vi "write_cred_xml.vi"() -> ()   [LabVIEW 2018]
uses:
  Ctrl/cred_ctrl.ctl
  Ctrl/cred_ip_info.ctl
  Ctrl/data_cred.ctl
  DataBase/MYsql/lv_mysql_connector_v1_lv8/typedefs/mysql_authentication.ctl
  <vilib>/NI/GXML/GXML.lvlib
panel:
  in  "database_inf":T1
  in  "database_ip":T2
  out "error out":errorcluster
  in  "XML File Path":path=path "C:/Users/prone/OneDrive/Documents/Acquire_MAP_copy-master/Acquire_MAP_copy-master/ignore/creds.xml"
  in  "error in":errorcluster
  in  "storage":T4
  out "XML String Out":string
  in  "slack":T4
  in  "database":T4
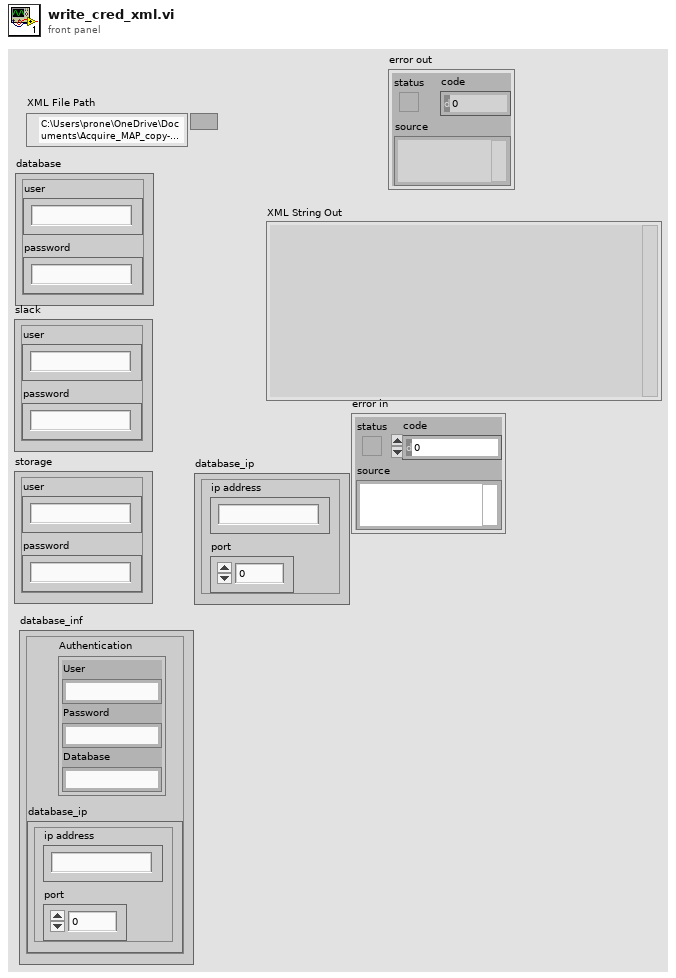
[diagram p1: front panel]
types:
  T1 = typedef "data_cred.ctl" = cluster{"database_ip":T2, "Authentication":T3}
  T2 = typedef "cred_ip_info.ctl" = cluster{"ip address":string, "port":dbl}
  T3 = typedef "mysql_authentication.ctl" = cluster{"User":string, "Password":string, "Database":string}
  T4 = typedef "cred_ctrl.ctl" = cluster{"user":string, "password":string}
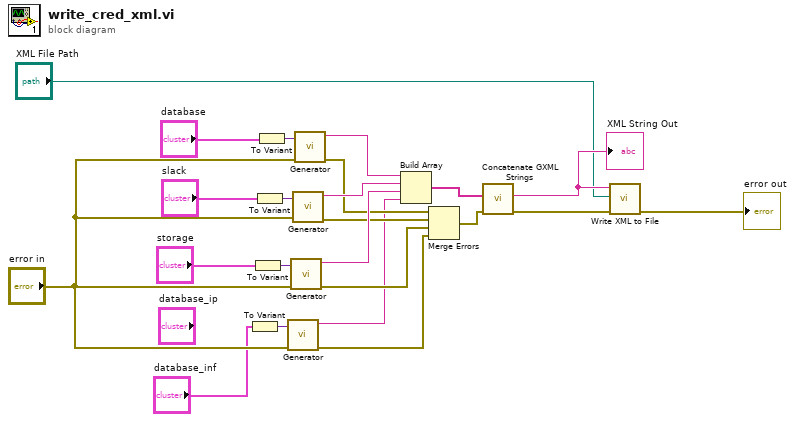
[diagram p0: block diagram]
diagram:
  n1 = To Variant(anything="database_inf") -> (Variant=w5:variant)
  n2 = To Variant(anything="storage") -> (Variant=w16:variant)
  n3 = To Variant(anything="slack") -> (Variant=w21:variant)
  n4 = To Variant(anything="database") -> (Variant=w23:variant)
  n5 = call <vilib>:"Generator.vi"("error in"="error in", "Variant"=w5) -> ("error out"=w3:errorcluster, "XML String Out"=w2:string)  [unwired: 8 in]
  n6 = call <vilib>:"Generator.vi"("error in"="error in", "Variant"=w16) -> ("error out"=w11:errorcluster, "XML String Out"=w14:string)  [unwired: 8 in]
  n7 = call <vilib>:"Generator.vi"("error in"="error in", "Variant"=w21) -> ("error out"=w12:errorcluster, "XML String Out"=w18:string)  [unwired: 8 in]
  n8 = call <vilib>:"Generator.vi"("error in"="error in", "Variant"=w23) -> ("error out"=w13:errorcluster, "XML String Out"=w19:string)  [unwired: 8 in]
  n9 = Build Array(w19, w18, w14, w2) -> (w17:string[])
  n10 = Merge Errors(w13, w12, w11, w3) -> (w10:errorcluster)
  n11 = call <vilib>:"Concatenate GXML Strings.vi"("error in"=w10, "GXML Strings"=w17) -> ("error out"=w8:errorcluster, "Concatenated GXML String"=w9:string)  [unwired: 8 in]
  "XML String Out" <- w9
  n12 = call <vilib>:"Write XML to File.vi"("error in"=w8, "XML File Path"="XML File Path", "XML Input"=w9) -> ("error out"=→"error out":errorcluster)  [unwired: 8 in]
